vi "TAT_Com_PLC.vi"() -> ()   [LabVIEW 2017]
uses:
  Controls/PLC_DATA_READ.ctl
  Controls/PLC_DATA_WRITE.ctl
  <vilib>/NI/Modbus Library/API/Wrapper/Create TCP Master.vi
  <vilib>/NI/Modbus Library/API/Master/Modbus Master.lvclass
  <vilib>/NI/Modbus Library/API/Wrapper/API Main.lvlib
panel:
  out "error out write":errorcluster
  out "error out read":errorcluster
  out "register values":u16[](array[numeric])
  out "error out":errorcluster
  in  "error in":errorcluster
  in  "stop":bool
  # "SCAN OK\nSCAN NG \nSoftware on Bit\nRQST FRM TCO REST SCN DT"
  # "STATION 1"
  # "1\tModel\t40202\tDecimal Numbers for Varient\n2\tJob Status\t40203\t1 for Ok & 0 for Not OK\n3\tSeq Status\t40204\tTo show SOP for Station 1 as per Varient\n4\tWeight\t40205\tDispensed Weight in Grams\n5\tReady Read\t40206\tSCADA will get 1 in this register after cycle complete (For printing purpose)"
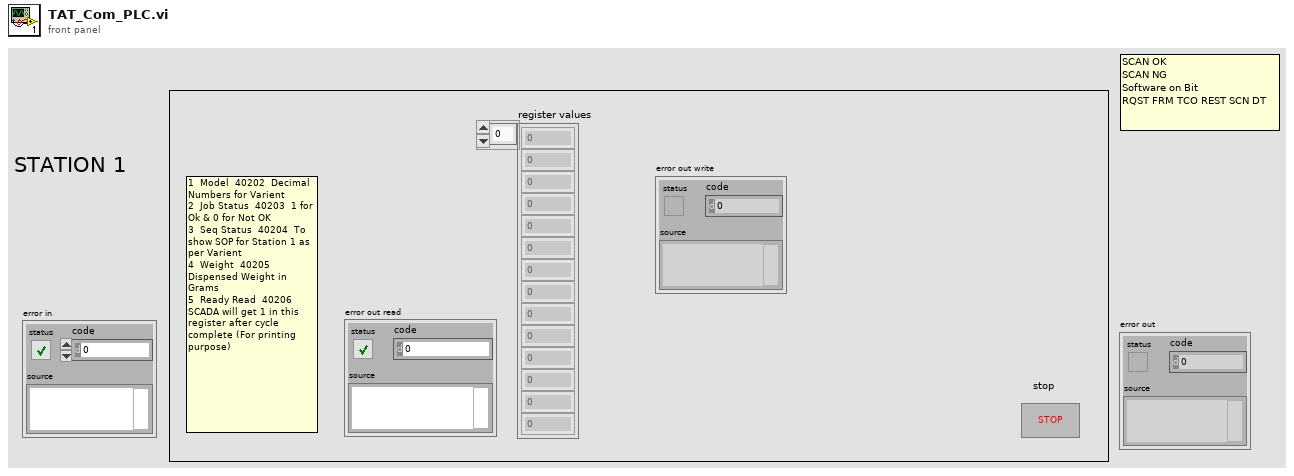
[diagram p1: front panel]
types:
  T1 = typedef "PLC_DATA_WRITE.ctl" = cluster{"Register to write":u16, "Labview to PLC Data":u16}
  T2 = typedef "PLC_DATA_READ.ctl" = cluster{"PLC to Labview Data":i32[], "Error Status in PLC Loop":errorcluster}
  T3 = enum32{"invalid app kind", "Development System", "Run Time System", "Student Edition", "Embedded LabVIEW", "Evaluation", "Custom"}
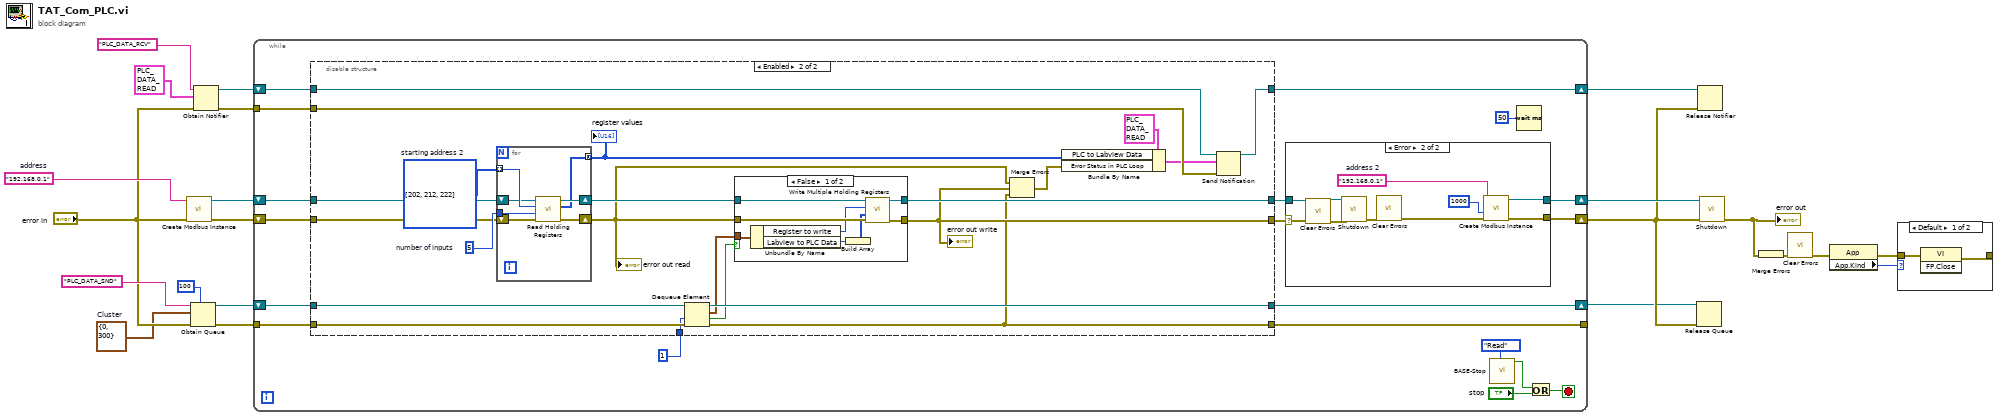
[diagram p0: block diagram]
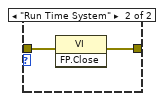
[diagram p5: hidden frame]
diagram:
  w6 = T1 {"Register to write"=0, "Labview to PLC Data"=300}  # Cluster
  w22 = "192.168.0.1"  # address
  n1 = call-poly <vilib>:"Create Modbus Instance.vi"("error in"="error in", "address"=w22) -> ("error out"=w15:errorcluster, "TCP master instance"=w14:refnum<class "Modbus Master.lvclass">)  [unwired: 8 in]
  n2 = Obtain Queue(max queue size (-1, unlimited)=100, name (unnamed)="PLC_DATA_SND", element data type=w6, error in (no error)="error in") -> (queue out=w4:refnum<queue>, error out=w3:errorcluster)  [unwired: 1 in, 1 out]
  n3 = Obtain Notifier(name (unnamed)="PLC_DATA_RCV", notification data type=T2 {"PLC to Labview Data"=[0, 0, 0, 0, 0, 0, 0, 0, 0, 0, 0, 0, 0, 0, 0], "Error Status in PLC Loop"={"status"=FALSE, "code"=0, "source"=""}}, error in (no error)="error in") -> (notifier out=w11:refnum<notifier>, error out=w12:errorcluster)  [unwired: 1 in, 1 out]
  n4 = while {
    shift-right: [w39] -> w21
    shift-left: w14 -> [w31]
    shift-right: [w38] -> w2
    shift-left: w15 -> [w32]
    tunnel: w12 -> [w28]
    shift-right: [w29] -> w10
    shift-left: w11 -> [w30]
    shift-right: [w25] -> w1
    shift-left: w4 -> [w27]
    tunnel: w3 -> [w26]
    tunnel: [w24] -> _
    stop <- w40 stop-if-true
    n5 = disable-structure shown="Enabled" {
      disable-tunnel: [w42 w54] -> w34
      disable-tunnel: [w43 w55] -> w33
      disable-tunnel: w32 -> [w42 w64]
      disable-tunnel: w31 -> [w43 w63]
      disable-tunnel: [w44 w61] -> w29
      disable-tunnel: w30 -> [w44 w62]
      disable-tunnel: w28 -> [_ w60]
      disable-tunnel: w27 -> [_ w51]
      disable-tunnel: w26 -> [_ w50]
      disable-tunnel: [_ w49] -> w25
      disable-tunnel: [_ w45] -> w24
      disable-tunnel: 1 ("timeout in ms (-1)") -> [_ w48]
      frame Disabled {
      }
      frame Enabled {
        w65 = u16 5  # number of inputs
        w66 = u16[] [202, 212, 222]  # starting address 2
        n6 = for {
          tunnel: w66 -> [w81] mode=indexing
          tunnel: w65 -> [w80]
          shift-right: [w82] -> w53
          shift-left: w64 -> [w79]
          shift-right: [w83] -> w56
          shift-left: w63 -> [w78]
          tunnel: [w77] -> w59 mode=concatenating
          n7 = call-dynamic "Read Holding Registers.vi"("error in"=w79, "number of inputs"=w80, "starting address"=w81, "Modbus master in"=w78) -> ("error out"=w82:errorcluster, "register values"=w77:u16[], "Modbus master out"=w83:refnum<class "Modbus Master.lvclass">)  [unwired: 5 in]
        }
        "register values" <- w59
        "error out read" <- w53
        n8 = Dequeue Element(queue=w51, timeout in ms (-1)=w48, error in (no error)=w50) -> (queue out=w49:refnum<queue>, element=w46:T1, timed out?=w47:bool, error out=w45:errorcluster)
        n9 = case shown="False" w47 {
          tunnel: w56 -> [w74 w76]
          tunnel: [w73 w76] -> w55
          tunnel: [w72 w75] -> w54
          tunnel: w53 -> [w71 w75]
          tunnel: w46 -> [w70 _]
          frame False {
            n10 = Unbundle By Name(w70) -> ("Register to write"=w69:u16, "Labview to PLC Data"=w68:u16)
            n11 = Build Array(w68) -> (w67:u16[])
            n12 = call-dynamic "Write Multiple Holding Registers.vi"("error in"=w71, "registers to write"=w67, "starting address"=w69, "Modbus master in"=w74) -> ("error out"=w72:errorcluster, "Modbus master out"=w73:refnum<class "Modbus Master.lvclass">)  [unwired: 6 in]
          }
          frame True {
          }
        }
        "error out write" <- w54
        n13 = Merge Errors(w53, w54, w45) -> (w52:errorcluster)
        n14 = Bundle By Name(cluster=T2 {"PLC to Labview Data"=[0, 0, 0, 0, 0, 0, 0, 0, 0, 0, 0, 0, 0, 0, 0], "Error Status in PLC Loop"={"status"=FALSE, "code"=0, "source"=""}}, "PLC to Labview Data"=w59, "Error Status in PLC Loop"=w52) -> (w58:T2)
        n15 = Send Notification(notification=w58, notifier=w62, error in (no error)=w60) -> (notifier out=w61:refnum<notifier>)  [unwired: 1 out]
      }
    }
    n16 = case shown="Error" w34 {
      selector: w34 -> [w84 w94]
      tunnel: w33 -> [w85 w92]
      tunnel: [w85 w88] -> w39
      tunnel: [w84 w87] -> w38
      frame No Error {
      }
      frame Error {
        w90 = "192.168.0.1"  # address 2
        n17 = call <vilib>:"Clear Errors.vi"("error in (no error)"=w94) -> ("error out"=w93:errorcluster)  [unwired: 5 in, 1 out]
        n18 = call-dynamic "Shutdown.vi"("error in"=w93, "Modbus master in"=w92) -> ("error out"=w91:errorcluster)  [unwired: 9 in]
        n19 = call <vilib>:"Clear Errors.vi"("error in (no error)"=w91) -> ("error out"=w89:errorcluster)  [unwired: 5 in, 1 out]
        n20 = call-poly <vilib>:"Create Modbus Instance.vi"("error in"=w89, "connect timeout ms"=1000, "address"=w90) -> ("error out"=w87:errorcluster, "TCP master instance"=w88:refnum<class "Modbus Master.lvclass">)  [unwired: 7 in]
      }
    }
    n21 = call "BASE-Stop.vi"("Enum"=enum16{"Read", "Write"}."Read") -> ("Stop"=w35:bool)  [unwired: 10 in]
    n22 = Wait (ms)(milliseconds to wait=u32 50) -> ()  [unwired: 1 out]
    n23 = Or(x=w35, y="stop") -> (x .or. y?=w40:bool)
  }
  n24 = Release Queue(queue=w1, error in (no error)=w2) -> ()  [unwired: 1 in, 3 out]
  n25 = Release Notifier(notifier=w10, error in (no error)=w2) -> ()  [unwired: 1 in, 3 out]
  n26 = call-dynamic "Shutdown.vi"("error in"=w2, "Modbus master in"=w21) -> ("error out"=w17:errorcluster)  [unwired: 9 in]
  "error out" <- w17
  n27 = Merge Errors(w17) -> (w16:errorcluster)
  n28 = call <vilib>:"Clear Errors.vi"("error in (no error)"=w16) -> ("error out"=w18:errorcluster)  [unwired: 5 in, 1 out]
  n29 = property class="App"(error in=w18) -> (error out=w19:errorcluster, "App.Kind"=w20:T3)  [unwired: 1 in, 1 out]
  n30 = case shown="Default" w20 {
    tunnel: w19 -> [w96 w98]
    tunnel: [w95 w97] -> _
    frame Default {
      n31 = invoke class="VI" method="FP.Close"(error in=w96) -> (error out=w95:errorcluster)  [unwired: 2 in, 2 out]
    }
    frame "Run Time System" {
      n32 = invoke class="VI" method="FP.Close"(error in=w98) -> (error out=w97:errorcluster)  [unwired: 2 in, 2 out]
    }
  }
